vi "Project Points.vi"(6 "Camera Parameters":T6, 8 "error in (no error)":errorcluster, 10 "Pose":T3, 11 "Object Points":T1[](array[typedef])) -> (0 "error out":errorcluster, 3 "Image Points":T2[](array[typedef]))   [LabVIEW 2020, in "ar.lvlib"]
doc: "Project object points into camera image points for a camera with the specified Pose and Camera Parameters."
uses:
  ar.lvlib
  common/Camera Parameters.ctl
  common/Camera Matrix.ctl
  common/Camera Distortion Coefficients.ctl
  Pose.ctl
  rvec.ctl
  tvec.ctl
  common/Image Point (Float).ctl
  common/Object Point (Float).ctl
  common/common.lvlib
  common/bin/gartoolkit_ar_32-1.dll
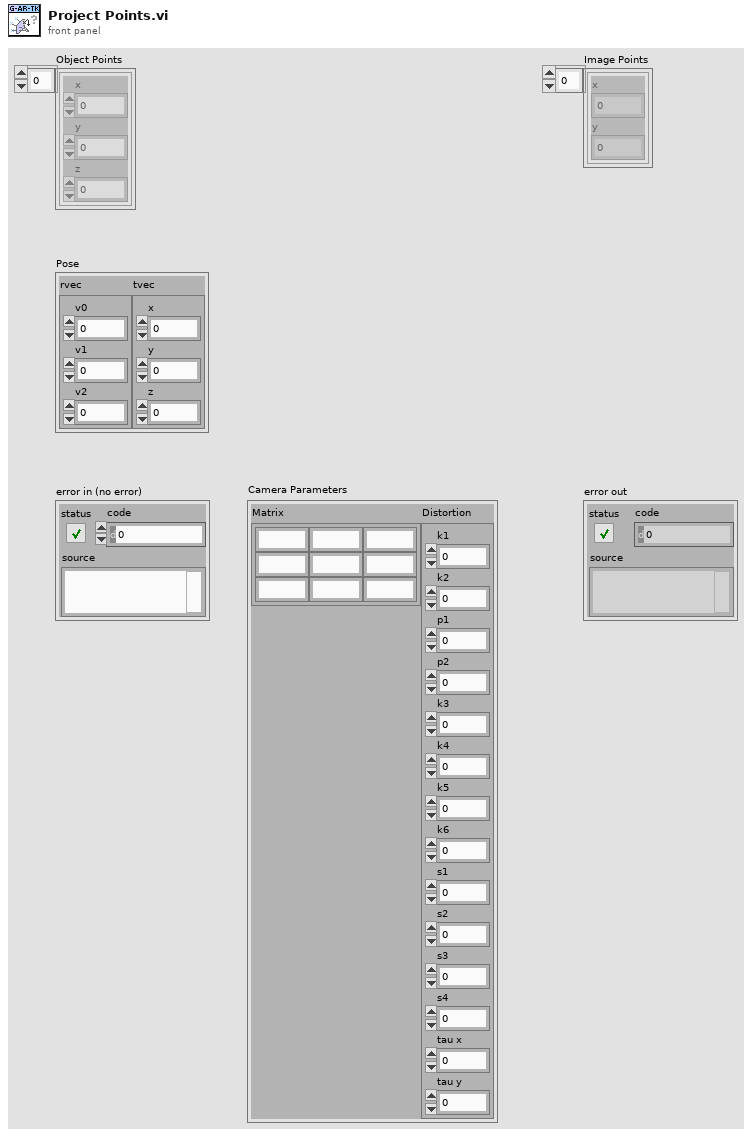
[diagram p1: front panel]
types:
  T1 = typedef "common.lvlib/Object Point (Float).ctl" = cluster{"x":dbl, "y":dbl, "z":dbl}
  T2 = typedef "common.lvlib/Image Point (Float).ctl" = cluster{"x":dbl, "y":dbl}
  T3 = typedef "ar.lvlib/Pose.ctl" = cluster{"rvec":T4, "tvec":T5}
  T4 = typedef "ar.lvlib/rvec.ctl" = cluster{"v0":dbl, "v1":dbl, "v2":dbl}
  T5 = typedef "ar.lvlib/tvec.ctl" = cluster{"x":dbl, "y":dbl, "z":dbl}
  T6 = typedef "common.lvlib/Camera Parameters.ctl" = cluster{"Matrix":T7, "Distortion":T8}
  T7 = typedef "common.lvlib/Camera Matrix.ctl" = cluster{"m 0,0":dbl, "m 0,1":dbl, "m 0,2":dbl, "m 1,0":dbl, "m 1,1":dbl, "m 1,2":dbl, "m 2,0":dbl, "m 2,1":dbl, "m 2,2":dbl}
  T8 = typedef "common.lvlib/Camera Distortion Coefficients.ctl" = cluster{"k1":dbl, "k2":dbl, "p1":dbl, "p2":dbl, "k3":dbl, "k4":dbl, "k5":dbl, "k6":dbl, "s1":dbl, "s2":dbl, "s3":dbl, "s4":dbl, "tau x":dbl, "tau y":dbl}
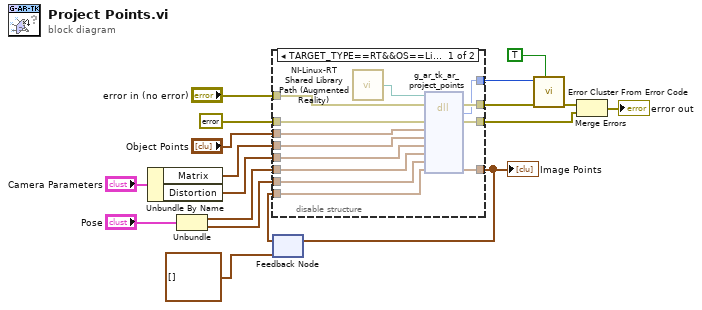
[diagram p0: block diagram]
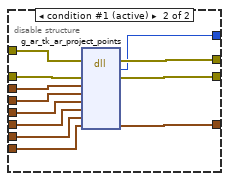
[diagram p2: hidden frame]
diagram:
  n1 = Unbundle By Name("Camera Parameters") -> ("Matrix"=w11:T7, "Distortion"=w10:T8)
  n2 = Unbundle("Pose") -> ("rvec"=w9:T4, "tvec"=w8:T5)
  n3 = feedback #1(T2[] [] ("Image Points")) -> (w2:T2[])
  n4 = disable-structure shown="TARGET_TYPE==RT&&OS==Linux" {
    disable-tunnel: "error in (no error)" -> [w31 w43]
    disable-tunnel: errorcluster {"status"=FALSE, "code"=0, "source"=""} ("error constant") -> [w30 w42]
    disable-tunnel: "Object Points" -> [w29 w41]
    disable-tunnel: w11 -> [w28 w40]
    disable-tunnel: w10 -> [w27 w39]
    disable-tunnel: w9 -> [w26 w38]
    disable-tunnel: w8 -> [w25 w37]
    disable-tunnel: w2 -> [w24 w36]
    disable-tunnel: [w23 w35] -> w7
    disable-tunnel: [w22 w34] -> w6
    disable-tunnel: [w21 w33] -> w5
    disable-tunnel: [w20 w32] -> w4
    frame condition #0 {
      n5 = call "NI-Linux-RT Shared Library Path (Augmented Reality).vi"() -> ("Path"=w19:path)
      n6 = dll-call lib="?" fn="g_ar_tk_ar_project_points" ("g_ar_toolkit.*.*:g_ar_tk_image_copy")(path in=w19, error in=w31, "error_cluster"=w30, "object_points"=w29, "camera_matrix"=w28, "camera_distortion"=w27, "rvec"=w26, "tvec"=w25, "image_points"=w24) -> (error out=w23:errorcluster, w22:i32, "error_cluster"=w21:errorcluster, "image_points"=w20:T2[])  [unwired: 6 in, 1 out]
    }
    frame condition #1 (active) {
      n7 = dll-call lib="C:/serenial/lib/g-augmented-reality-toolkit/LabVIEW/common/bin/gartoolkit_ar_*-1.*" fn="g_ar_tk_ar_project_points" ("g_ar_toolkit.*.*:g_ar_tk_image_copy")(error in=w43, "error_cluster"=w42, "object_points"=w41, "camera_matrix"=w40, "camera_distortion"=w39, "rvec"=w38, "tvec"=w37, "image_points"=w36) -> (error out=w35:errorcluster, w34:i32, "error_cluster"=w33:errorcluster, "image_points"=w32:T2[])  [unwired: 7 in, 1 out]
    }
  }
  "Image Points" <- w4
  n8 = feedback-in #1(w4) -> ()
  n9 = call <vilib>:"Error Cluster From Error Code.vi"("show call chain? (False)"=TRUE, "error in (no error)"=w7, "error code (0)"=w6) -> ("error out"=w18:errorcluster)  [unwired: 6 in]
  n10 = Merge Errors(w18, w5) -> (→"error out":errorcluster)
